vi "IT-M3400 LIST_Output.vi"() -> ()   [LabVIEW 2015]
doc: "The main function of the example is to set the parameters of the list under the voltage type of the source mode and run it"
uses:
  <instrlib>/IT-M3400/IT-M3400.lvlib
panel:
  in  "Serial Configuration":T1={"Baud Rate"=9600, "Parity"=0, "Data Bits"=8, "Stop Bits"=10, "Flow Control"=0} {"Flow Control" items=["None", "XON/XOFF", "RTS/CTS", "XON/XOFF & RTS/CTS", "DTR/DSR", "XON/XOFF & DTR/DSR"]; "Stop Bits" items=["1.0"=10, "1.5"=15, "2.0"=20]; "Data Bits" items=["7"=7, "8"=8]; "Parity" items=["None", "Odd", "Even", "Mark", "Space"]; "Baud Rate" items=["300"=300, "600"=600, "1200"=1200, "2400"=2400, "4800"=4800, "9600"=9600, "19200"=19200]}
  in  "Terminate Type":u8(ring) items=["Normal", "Last"]
  in  "Current limit -(A)":dbl
  in  "Current limit+(A)":dbl
  in  "Save File(1-10)":u8=1 min=1 max=10 step=1
  in  "Slew":dbl[](array[numeric])
  in  "Width(S)":dbl[](array[numeric])
  in  "Voltage(V)":dbl[](array[numeric])
  in  "Repeat":u32=1 min=1 step=1
  in  "Step Count":u8=1 min=1 max=100 step=1
  in  "Channel":i32(ring)=1 items=["Channel 1"=1, "Channel 2"=2, "Channel 3"=3, "Channel 4"=4, "Channel 5"=5, "Channel 6"=6, "Channel 7"=7, "Channel 8"=8, "Channel 8"=9, "Channel 10"=10, "Channel 11"=11, "Channel 12"=12, "Channel 13"=13, "Channel 14"=14, "Channel 15"=15, "Channel 16"=16]
  in  "VISA resource name":refnum<visa-resource-name>
  # "List Function"
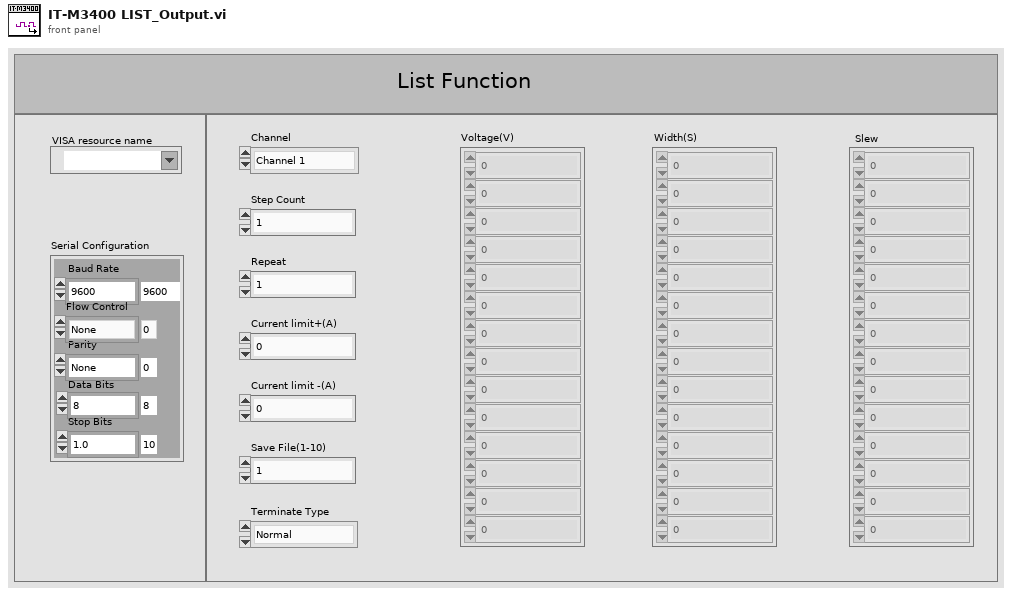
[diagram p1: front panel]
types:
  T1 = cluster{"Baud Rate":u32, "Parity":u16, "Data Bits":u16, "Stop Bits":u16, "Flow Control":u16}
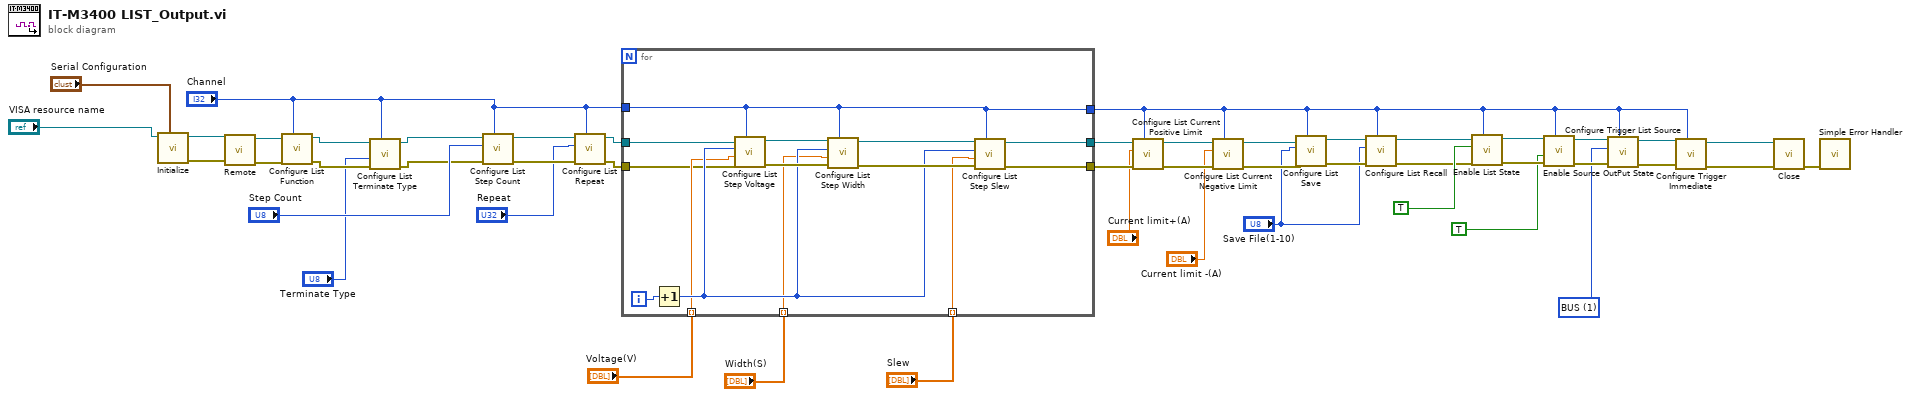
[diagram p0: block diagram]
diagram:
  w33 = u8 1 items=["KEYPad", "BUS"] ("Ponsetup Type(0:Keypad)")
  n1 = call <instrlib>:"Initialize.vi"("Serial Configuration"="Serial Configuration", "VISA resource name"="VISA resource name") -> ("error out"=w12:errorcluster, "VISA resource name out"=w13:refnum<visa-resource-name>)  [unwired: 8 in]
  n2 = call <instrlib>:"Remote.vi"("error in"=w12, "VISA resource name"=w13) -> ("error out"=w47:errorcluster, "VISA resource name out"=w46:refnum<visa-resource-name>)  [unwired: 8 in]
  n3 = call <instrlib>:"Configure List Function.vi"("Channel"="Channel", "error in"=w47, "VISA resource name"=w46) -> ("error out"=w9:errorcluster, "VISA resource name out"=w10:refnum<visa-resource-name>)  [unwired: 7 in]
  n4 = call <instrlib>:"Configure List Terminate Type.vi"("VISA resource name"=w10, "Terminate Type"="Terminate Type", "error in"=w9, "Channel"="Channel") -> ("VISA resource name out"=w8:refnum<visa-resource-name>, "error out"=w7:errorcluster)  [unwired: 5 in]
  n5 = call <instrlib>:"Configure List Step Count.vi"("Channel"="Channel", "error in"=w7, "Step Count"="Step Count", "VISA resource name"=w8) -> ("error out"=w43:errorcluster, "VISA resource name out"=w44:refnum<visa-resource-name>)  [unwired: 6 in]
  n6 = call <instrlib>:"Configure List Repeat.vi"("Channel"="Channel", "error in"=w43, "Repeat"="Repeat", "VISA resource name"=w44) -> ("error out"=w24:errorcluster, "VISA resource name out"=w25:refnum<visa-resource-name>)  [unwired: 6 in]
  n7 = for {
    tunnel: "Channel" -> [w48]
    tunnel: "Voltage(V)" -> [w55] mode=indexing
    tunnel: "Width(S)" -> [w54] mode=indexing
    tunnel: "Slew" -> [w53] mode=indexing
    tunnel: [w48] -> w17
    tunnel: w25 -> [w50]
    tunnel: [w52] -> w23
    tunnel: w24 -> [w49]
    tunnel: [w51] -> w22
    i -> [w57]
    n8 = Increment(x=w57) -> (x+1=w56:i32)
    n9 = call <instrlib>:"Configure List Step Voltage.vi"("Channel"=w48, "error in"=w49, "Voltage(V)"=w55, "Step"=w56, "VISA resource name"=w50) -> ("error out"=w60:errorcluster, "VISA resource name out"=w61:refnum<visa-resource-name>)  [unwired: 5 in]
    n10 = call <instrlib>:"Configure List Step Width.vi"("Channel"=w48, "error in"=w60, "Width(S)"=w54, "Step"=w56, "VISA resource name"=w61) -> ("error out"=w59:errorcluster, "VISA resource name out"=w58:refnum<visa-resource-name>)  [unwired: 5 in]
    n11 = call <instrlib>:"Configure List Step Slew.vi"("Channel"=w48, "error in"=w59, "Slew"=w53, "Step"=w56, "VISA resource name"=w58) -> ("error out"=w51:errorcluster, "VISA resource name out"=w52:refnum<visa-resource-name>)  [unwired: 5 in]
  }
  n12 = call <instrlib>:"Configure List Current Positive Limit.vi"("Channel"=w17, "error in"=w22, "Limit(A)"="Current limit+(A)", "VISA resource name"=w23) -> ("error out"=w20:errorcluster, "VISA resource name out"=w21:refnum<visa-resource-name>)  [unwired: 6 in]
  n13 = call <instrlib>:"Configure List Current Negative Limit.vi"("Channel"=w17, "error in"=w20, "Limit(A)"="Current limit -(A)", "VISA resource name"=w21) -> ("error out"=w18:errorcluster, "VISA resource name out"=w19:refnum<visa-resource-name>)  [unwired: 6 in]
  n14 = call <instrlib>:"Configure List Save.vi"("Channel"=w17, "error in"=w18, "File"="Save File(1-10)", "VISA resource name"=w19) -> ("error out"=w31:errorcluster, "VISA resource name out"=w32:refnum<visa-resource-name>)  [unwired: 6 in]
  n15 = call <instrlib>:"Configure List Recall.vi"("Channel"=w17, "error in"=w31, "File"="Save File(1-10)", "VISA resource name"=w32) -> ("error out"=w29:errorcluster, "VISA resource name out"=w30:refnum<visa-resource-name>)  [unwired: 6 in]
  n16 = call <instrlib>:"Enable List State.vi"("Channel"=w17, "error in"=w29, "State"=TRUE ("list状态控制"), "VISA resource name"=w30) -> ("error out"=w39:errorcluster, "VISA resource name out"=w40:refnum<visa-resource-name>)  [unwired: 6 in]
  n17 = call <instrlib>:"Enable Source OutPut State.vi"("Channel"=w17, "error in"=w39, "State"=TRUE ("ON\\OFF"), "VISA resource name"=w40) -> ("error out"=w36:errorcluster, "VISA resource name out"=w37:refnum<visa-resource-name>)  [unwired: 6 in]
  n18 = call <instrlib>:"Configure Trigger List Source.vi"("Channel"=w17, "error in"=w36, "Type"=w33, "VISA resource name"=w37) -> ("error out"=w34:errorcluster, "VISA resource name out"=w35:refnum<visa-resource-name>)  [unwired: 6 in]
  n19 = call <instrlib>:"Configure Trigger Immediate.vi"("Channel"=w17, "error in"=w34, "VISA resource name"=w35) -> ("error out"=w1:errorcluster, "VISA resource name out"=w2:refnum<visa-resource-name>)  [unwired: 7 in]
  n20 = call <instrlib>:"Close.vi"("error in"=w1, "VISA resource name"=w2) -> ("error out"=w3:errorcluster)  [unwired: 9 in]
  n21 = call <vilib>:"Simple Error Handler.vi"("error in (no error)"=w3) -> ()  [unwired: 4 in, 5 out]
